vi "Test.vi"() -> ()   [LabVIEW 2024]
uses:
  State Machine/State Machine/State Machine.lvclass
  C:/Program Files (x86)/National Instruments/LabVIEW 2024/vi.lib/ActorFramework/Actor/Actor.lvclass
  <vilib>/ActorFramework/Message Enqueuer/Message Enqueuer.lvclass/Message Enqueuer.ctl
  <vilib>/ActorFramework/Message Enqueuer/Enqueue.vi
  State Machine/State Machine Messages/Start Cycle Msg/Start Cycle Msg.lvclass
  C:/Program Files (x86)/National Instruments/LabVIEW 2024/vi.lib/ActorFramework/Message/Message.lvclass
  State Machine/State Machine Messages/Logging Stopped Msg/Logging Stopped Msg.lvclass
  State Machine/State Machine Messages/Cycle Complete Msg/Cycle Complete Msg.lvclass
  <vilib>/ActorFramework/Stop Msg/Stop Msg.lvclass
  <vilib>/ActorFramework/Message Priority Queue/Priority Enqueue.vi
  <vilib>/ActorFramework/Actor/Actor.lvclass
  State Machine/State Machine Messages/Start Logging Msg/Start Logging Msg.lvclass
  C:/Users/uspoaotto/OneDrive - Oregon Tool/Desktop/working copies/stateMachineActor/src/State Machine/State Machine/State Machine.lvclass
panel:
  in  "Start Logging":bool
  in  "Logging Stopped":bool
  in  "Stop":bool
  in  "Cycle Complete":bool
  in  "Start Cycle":bool
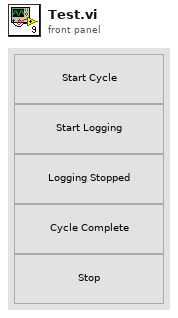
[diagram p1: front panel]
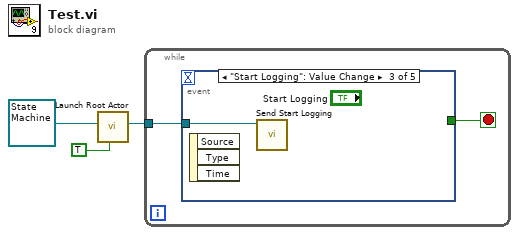
[diagram p0: block diagram]
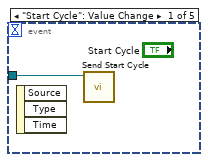
[diagram p2: hidden frame]
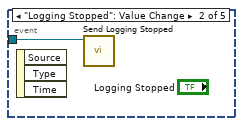
[diagram p3: hidden frame]
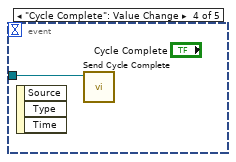
[diagram p4: hidden frame]
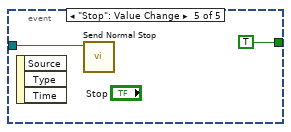
[diagram p5: hidden frame]
diagram:
  n1 = call <vilib>:"Launch Root Actor.vi"("Open Actor Core front panel? (F)"=TRUE, "Actor"=refnum<class "State Machine.lvclass"> refnum ("State Machine.lvlib:State Machine.lvclass")) -> ("Actor's Enqueuer"=w2:refnum<class "Message Enqueuer.lvclass">)  [unwired: 8 in, 1 out]
  n2 = while {
    tunnel: w2 -> [w4]
    stop <- w5 stop-if-true
    n3 = event shown="[2] \"Start Logging\": Value Change" {
      selector: _ -> [_ _ _ _ _]
      dyn-events: _ -> [_ _ _ _ _]
      timeout: _ -> [_ _ _ _ _]
      tunnel: w4 -> [w6 w7 w8 w9 w11]
      tunnel: [_ _ _ _ TRUE] -> w5
      event "Start Cycle": Value Change {
        n4 = event-data() -> ()  [unwired: 1 in, 3 out]
        n5 = call "Send Start Cycle.vi"("Message Enqueuer"=w6) -> ()  [unwired: 9 in, 2 out]
      }
      event "Logging Stopped": Value Change {
        n6 = event-data() -> ()  [unwired: 1 in, 3 out]
        n7 = call "Send Logging Stopped.vi"("Message Enqueuer"=w7) -> ()  [unwired: 9 in, 2 out]
      }
      event "Start Logging": Value Change {
        n8 = event-data() -> ()  [unwired: 1 in, 3 out]
        n9 = call "Send Start Logging.vi"("Message Enqueuer"=w8) -> ()  [unwired: 9 in, 2 out]
      }
      event "Cycle Complete": Value Change {
        n10 = event-data() -> ()  [unwired: 1 in, 3 out]
        n11 = call "Send Cycle Complete.vi"("Message Enqueuer"=w9) -> ()  [unwired: 9 in, 2 out]
      }
      event "Stop": Value Change {
        n12 = event-data() -> ()  [unwired: 1 in, 3 out]
        n13 = call <vilib>:"Send Normal Stop.vi"("Message Enqueuer"=w11) -> ()  [unwired: 10 in, 1 out]
      }
    }
  }
